vi "fs_mm_converter.vi"(2 "mm in":dbl[](array[numeric]), 3 "fs in":dbl[](array[numeric])) -> (0 "mm out":dbl[](array[numeric]), 1 "fs out":dbl[](array[numeric]))   [LabVIEW 2019]
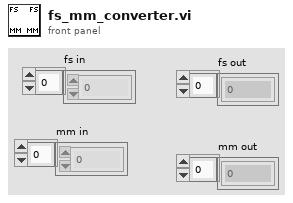
[diagram p1: front panel]
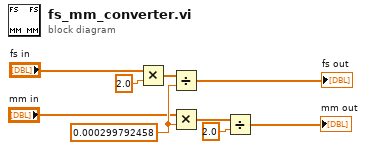
[diagram p0: block diagram]
diagram:
  w5 = 0.000299792458 ("y")
  n1 = Multiply(x="fs in", y=2.0) -> (x*y=w8:dbl[])
  n2 = Divide(x=w8, y=w5) -> (x/y=→"fs out":dbl[])
  n3 = Multiply(x="mm in", y=w5) -> (x*y=w7:dbl[])
  n4 = Divide(x=w7, y=2.0) -> (x/y=→"mm out":dbl[])
